vi "Init.vi"(8 "error in (no error)":errorcluster, 10 "Instrument String":variant, 11 "Chroma 19020":refnum<class "Chroma 190020.lvclass">) -> (0 "error out":errorcluster, 2 "Found?":bool=TRUE, 3 "Chroma 19020 out":refnum<class "Chroma 190020.lvclass">)   [LabVIEW 2025, in "HiPOT.lvlib" / "Chroma 190020.lvclass"]
uses:
  Chroma 190020.lvclass
  C:/Working copy/tss/Plugin/Engines/HiPOT/HiPOT Instrument/HiPOT Instrument.lvclass
  HiPOT configuration/HiPOT configuration.lvclass
  C:/Users/Public/Documents/Sandia National Labs/TSS Plugin/Abstract Engine.lvlibp/Instrument configuration/Instrument configuration.lvclass
  Chroma 190020.lvclass/Chroma 190020.ctl
  Users/Public/Documents/Sandia National Labs/TSS Plugin/Abstract Engine.lvlibp/Instrument configuration/Read Instrument Setting.vi
  Users/Public/Documents/Sandia National Labs/TSS Plugin/CEF.lvlibp/serializable configuration/CEF_serializable configuration.lvclass
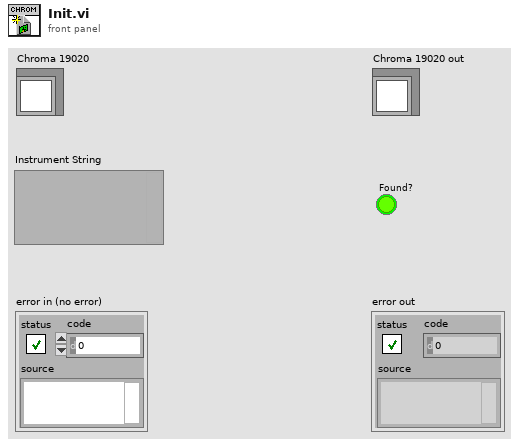
[diagram p1: front panel]
types:
  T1 = typedef "Abstract Engine.lvlibp/Instrument configuration.lvclass/Default Instrument.ctl" = cluster{"Type":string, "Address":string, "SW Alias":string, "Description":string, "Enabled":bool}
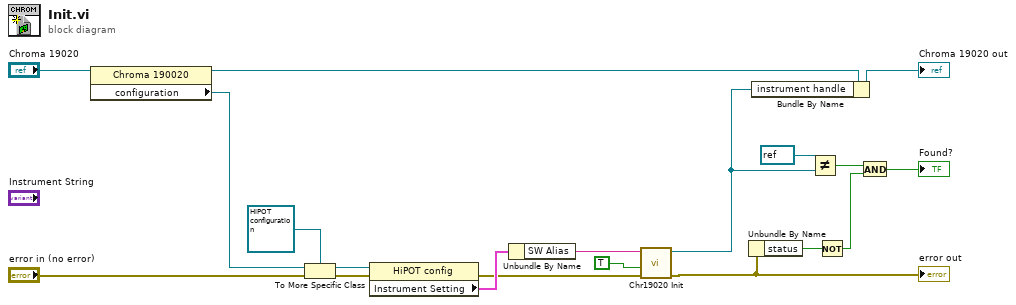
[diagram p0: block diagram]
diagram:
  n1 = property class="Chroma 190020"(reference="Chroma 19020") -> (reference out=w17:refnum<class "Chroma 190020.lvclass">, "configuration"=w10:refnum<class "CEF_serializable configuration.lvclass">)  [unwired: 1 in, 1 out]
  n2 = To More Specific Class(target class=refnum<class "HiPOT configuration.lvclass"> refnum ("ACIR.lvlib:ACIR config"), reference=w10, error in="error in (no error)") -> (specific class reference=w11:refnum<class "HiPOT configuration.lvclass">, error out=w12:errorcluster)
  n3 = property class="HiPOT config"(reference=w11, error in=w12) -> (error out=w5:errorcluster, "Instrument Setting"=w7:T1)  [unwired: 1 out]
  n4 = Unbundle By Name(w7) -> ("SW Alias"=w4:string)
  n5 = call <instrlib>:"Chr19020 Init.vi"("error in (no error)"=w5, "reset device"=TRUE, "resource name"=w4) -> ("error out"=w1:errorcluster, "instrument handle out"=w2:refnum<k15>)  [unwired: 7 in]
  "error out" <- w1
  n6 = Unbundle By Name(w1) -> ("status"=w16:bool)
  n7 = Bundle By Name(cluster=w17, "instrument handle"=w2) -> (→"Chroma 19020 out":refnum<class "Chroma 190020.lvclass">)
  n8 = Not Equal?(x=refnum<k15> refnum ("instrument handle"), y=w2) -> (x != y?=w14:bool)
  n9 = Not(x=w16) -> (.not. x?=w15:bool)
  n10 = And(x=w14, y=w15) -> (x .and. y?=→"Found?":bool)
